vi "HardwareConfiguration.vi"() -> (3 "configured?":bool=TRUE)   [LabVIEW 2018]
uses:
  InstrControl/InstrumentSetup.vi
  globals/QC_RunInformation.vi
  InstrControl/InstrControl.lvclass
panel:
  in  "Matrix Configurations":bool
  in  "Defaults Multimeter":bool
  in  "Multimeter":enum32{"Keithley 2000"}(tab)
  in  "Range Value\n(0.1 - 100)":dbl=100.0 format="%#.2g"
  in  "Range":u16(ring) items=["Auto", "Manual"]
  in  "Function":u16(ring)=3 items=["AC Current", "DC Current", "AC Voltage", "DC Voltage", "2W-Resistance", "4W-Resistance", "Period", "Frequency", "Temperature", "Diode", "Continuity"]
  in  "Address KE2000":refnum<visa-resource-name>="GPIB0::19::INSTR"
  in  "Defaults LCR":bool
  in  "LCRs":T1(tab)=enum."HP4284A"
  in  "AC frequency [Hz]":i32=1000 format="%#.3p"
  in  "RC Configuration":u16(ring) items=["serial", "parallel"]
  in  "AC amplitude [V]":sgl=0.1
  in  "Address WK6440B":refnum<visa-resource-name>="GPIB0::6::INSTR"
  in  "Address WK6425":refnum<visa-resource-name>
  in  "AC amplitude [V] WK6425":sgl=0.1 caption="AC amplitude [V]"
  in  "RC Configuration WK6425":u16(ring) caption="RC Configuration" items=["serial", "parallel"]
  in  "AC frequency [Hz] WK6425":i32=1000 caption="AC frequency [Hz]" format="%#.3p"
  in  "Address HP4284A":refnum<visa-resource-name>="GPIB0::13::INSTR"
  in  "AC amplitude [V] HP4284A":sgl=0.1 caption="AC amplitude [V]"
  in  "AC frequency [Hz] HP4284A":i32=1000 caption="AC frequency [Hz]" format="%#.3p"
  in  "RC Configuration HP4284A":u16(ring)=6 caption="RC Configuration" items=["CPD", "CPQ", "CPG", "CPRP", "CSD", "CSQ", "CSRS", "LPQ", "LPD", "LPG", "LPRP", "LSD", "LSQ", "LSRS", "RX", "ZTD", "ZTR", "GB", "YTD", "YTR"]
  in  "Consider OC":bool
  in  "Consider SC":bool
  in  "VISA address":refnum<visa-resource-name>="COM24" caption="Arduino address"
  out "Programm uploaded?":string="Make sure programme is uploaded to Arduino Uno ->"
  in  "Blank Button":bool
  in  "Supplies":T2(tab)=enum."Keithley 237"
  in  "Current Limit [µA]":sgl=100.0
  in  "Address KE2410":refnum<visa-resource-name>="GPIB0::16::INSTR"
  in  "Address KE487":refnum<visa-resource-name>
  in  "Compliance":u16(ring) items=["20µA", "2mA"]
  in  "Range:":u16(ring) items=["Autorange", "2nA", "20nA", "200nA", "2 microAmp", "20 microAmp", "200 microAmp", "2 milliAmp"]
  in  "Current Limit":u16(ring)=1 items=["OFF", "ON"]
  in  "Address KE6517":refnum<visa-resource-name>
  in  "current compliance \nlevel [mA]":dbl=0.0001 format="%.4f"
  in  "compliance/measurement\nrange (auto:0)":u16(ring)=6 items=["auto / auto", "1 nA / 1.1 V", "10 nA / 11 V", "100 nA / 110 V", "0.001 mA / 110 V", "0.01 mA / 110 V", "0.1 mA / 110 V", "1 mA / 110 V", "10 mA / 110 V", "100 mA / 110 V"]
  in  "Address KE236":refnum<visa-resource-name>
  in  "Address KE237":refnum<visa-resource-name>="GPIB0::16::INSTR"
  in  "current compliance \nlevel [uA] K237":dbl=30.0 caption="current compliance\nlevel [uA]" format="%.4f"
  in  "compliance/measurement\nrange (auto:0) K237":u16(ring)=6 caption="compliance/measurement\nrange (auto:0)" items=["auto / auto", "1 nA / 1.1 V", "10 nA / 11 V", "100 nA / 110 V", "1 uA / 1100 V", "10 uA / *", "100 uA / *", "1 mA / *", "10 mA / *", "100 mA / *"]
  in  "Defaults Supply":bool
  in  "OK Button":bool
  # "Hardware Configuration"
  # "Multimeter Configuration"
  # "Supply Configuration"
  # "Arduino Configuration"
  # "LCR Configuration"
  # "(Only for initialisation)"
  # "(Only for initialisation)"
  # "(Only for initialisation)"
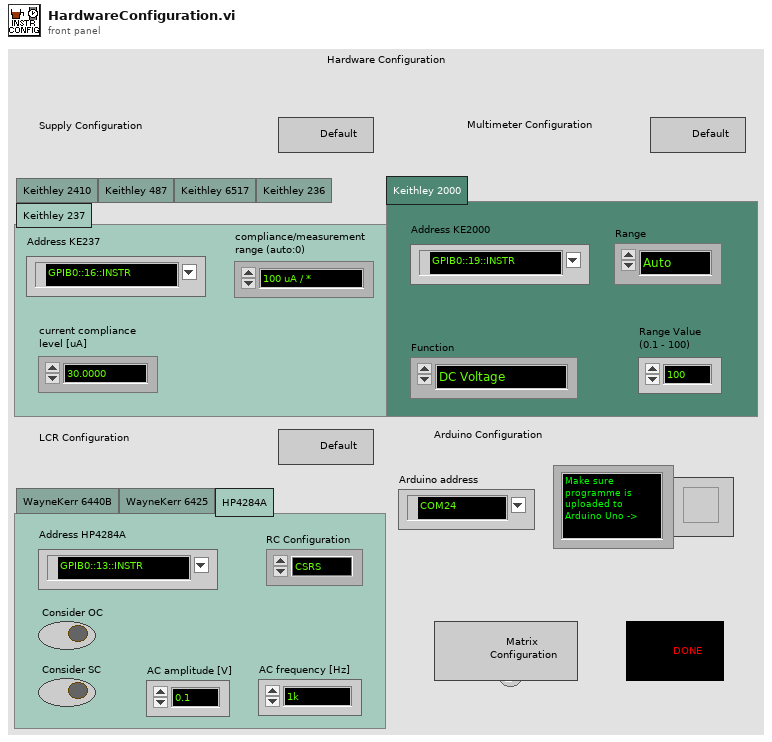
[diagram p1: front panel]
types:
  T1 = enum32{"WayneKerr 6440B", "WayneKerr 6425", "HP4284A"}
  T2 = enum32{"Keithley 2410", "Keithley 487", "Keithley 6517", "Keithley 236", "Keithley 237"}
  T3 = enum16{"CPD", "CPQ", "CPG", "CPRP", "CSD", "CSQ", "CSRS", "LPQ", "LPD", "LPG", "LPRP", "LSD", "LSQ", "LSRS", "RX", "ZTD", "ZTR", "GB", "YTD", "YTR"}
  T4 = cluster{"KE 2410":cluster{"Instrument name":string, "address":refnum<visa-resource-name>, "Instrument type":u16}, "KE 6517":cluster{"Instrument name":string, "address":refnum<visa-resource-name>, "Instrument type":u16}, "KE 487":cluster{"Instrument name":string, "address":refnum<visa-resource-name>, "Instrument type":u16}, "KE 236":cluster{"Instrument name":string, "address":refnum<visa-resource-name>, "Instrument type":u16}, "WK 6440B":cluster{"Instrument name":string, "address":refnum<visa-resource-name>, "Instrument type":u16}, "WK 6425":cluster{"Instrument name":string, "address":refnum<visa-resource-name>, "Instrument type":u16}, "Pickering Matrix":cluster{"Instrument name":string, "address":refnum<visa-resource-name>, "Instrument type":u16}, "KE 2000":cluster{"Instrument name":string, "address":refnum<visa-resource-name>, "Instrument type":u16}, "KE3706A Switching":cluster{"Instrument name":string, "address":refnum<visa-resource-name>, "Instrument type":u16}, "HP 4284A":cluster{"Instrument name":string, "address":refnum<visa-resource-name>, "Instrument type":u16}, "KE237":cluster{"Instrument name":string, "address":refnum<visa-resource-name>, "Instrument type":u16}}
  T5 = cluster{"VISA address":refnum<visa-resource-name>, "T sensor":enum16{"SHT", "DS"}, "Arduino":refnum<class "ArduinoControl.lvclass">}
  T6 = cluster{"Range":u16, "Range Value":dbl, "Function":u16, "KE2000":refnum<class "KE2000.lvclass">}
  T7 = cluster{"Current Limit":sgl, "KE2410":refnum<class "KE2410.lvclass">}
  T8 = cluster{"Compliance":u16, "Range:":u16, "KE487":refnum<class "KE487.lvclass">}
  T9 = cluster{"Current Limit":u16, "KE6517":refnum<class "KE6517.lvclass">}
  T10 = cluster{"current \ncompliance level":dbl, "compliance/\nmeasurement range (auto:0)":u16, "KE236":refnum<class "KE236.lvclass">}
  T11 = cluster{"current \ncompliance level":dbl, "compliance/\nmeasurement range (auto:0)":u16, "KE237":refnum<class "KE237.lvclass">}
  T12 = cluster{"Sensor Serial No.:":string, "Wafer Serial No.:":string, "Batch:":string, "Manufacturer:":string, "Device Category:":string, "Database Serial No.:":string, "Date Initiated:":string, "Time Initiated:":string, "Test":string, "Instruments used:":string, "Probeplan used:":string, "End of Run comment:":string, "User:":string}
  T13 = cluster{"RC Configuration":u16, "AC amplitude [V]":dbl, "AC frequency [Hz]":i32, "WK6440B":refnum<class "WK6440B.lvclass">}
  T14 = cluster{"RC Configuration":u16, "AC amplitude [V]":dbl, "AC frequency [Hz]":i32, "WK6425":refnum<class "WK6425.lvclass">}
  T15 = cluster{"RC Configuration":u16, "AC amplitude [V]":dbl, "Consider OC":bool, "Consider SC":bool, "AC frequency [Hz]":i32, "HP4284A":refnum<class "HP4284A.lvclass">}
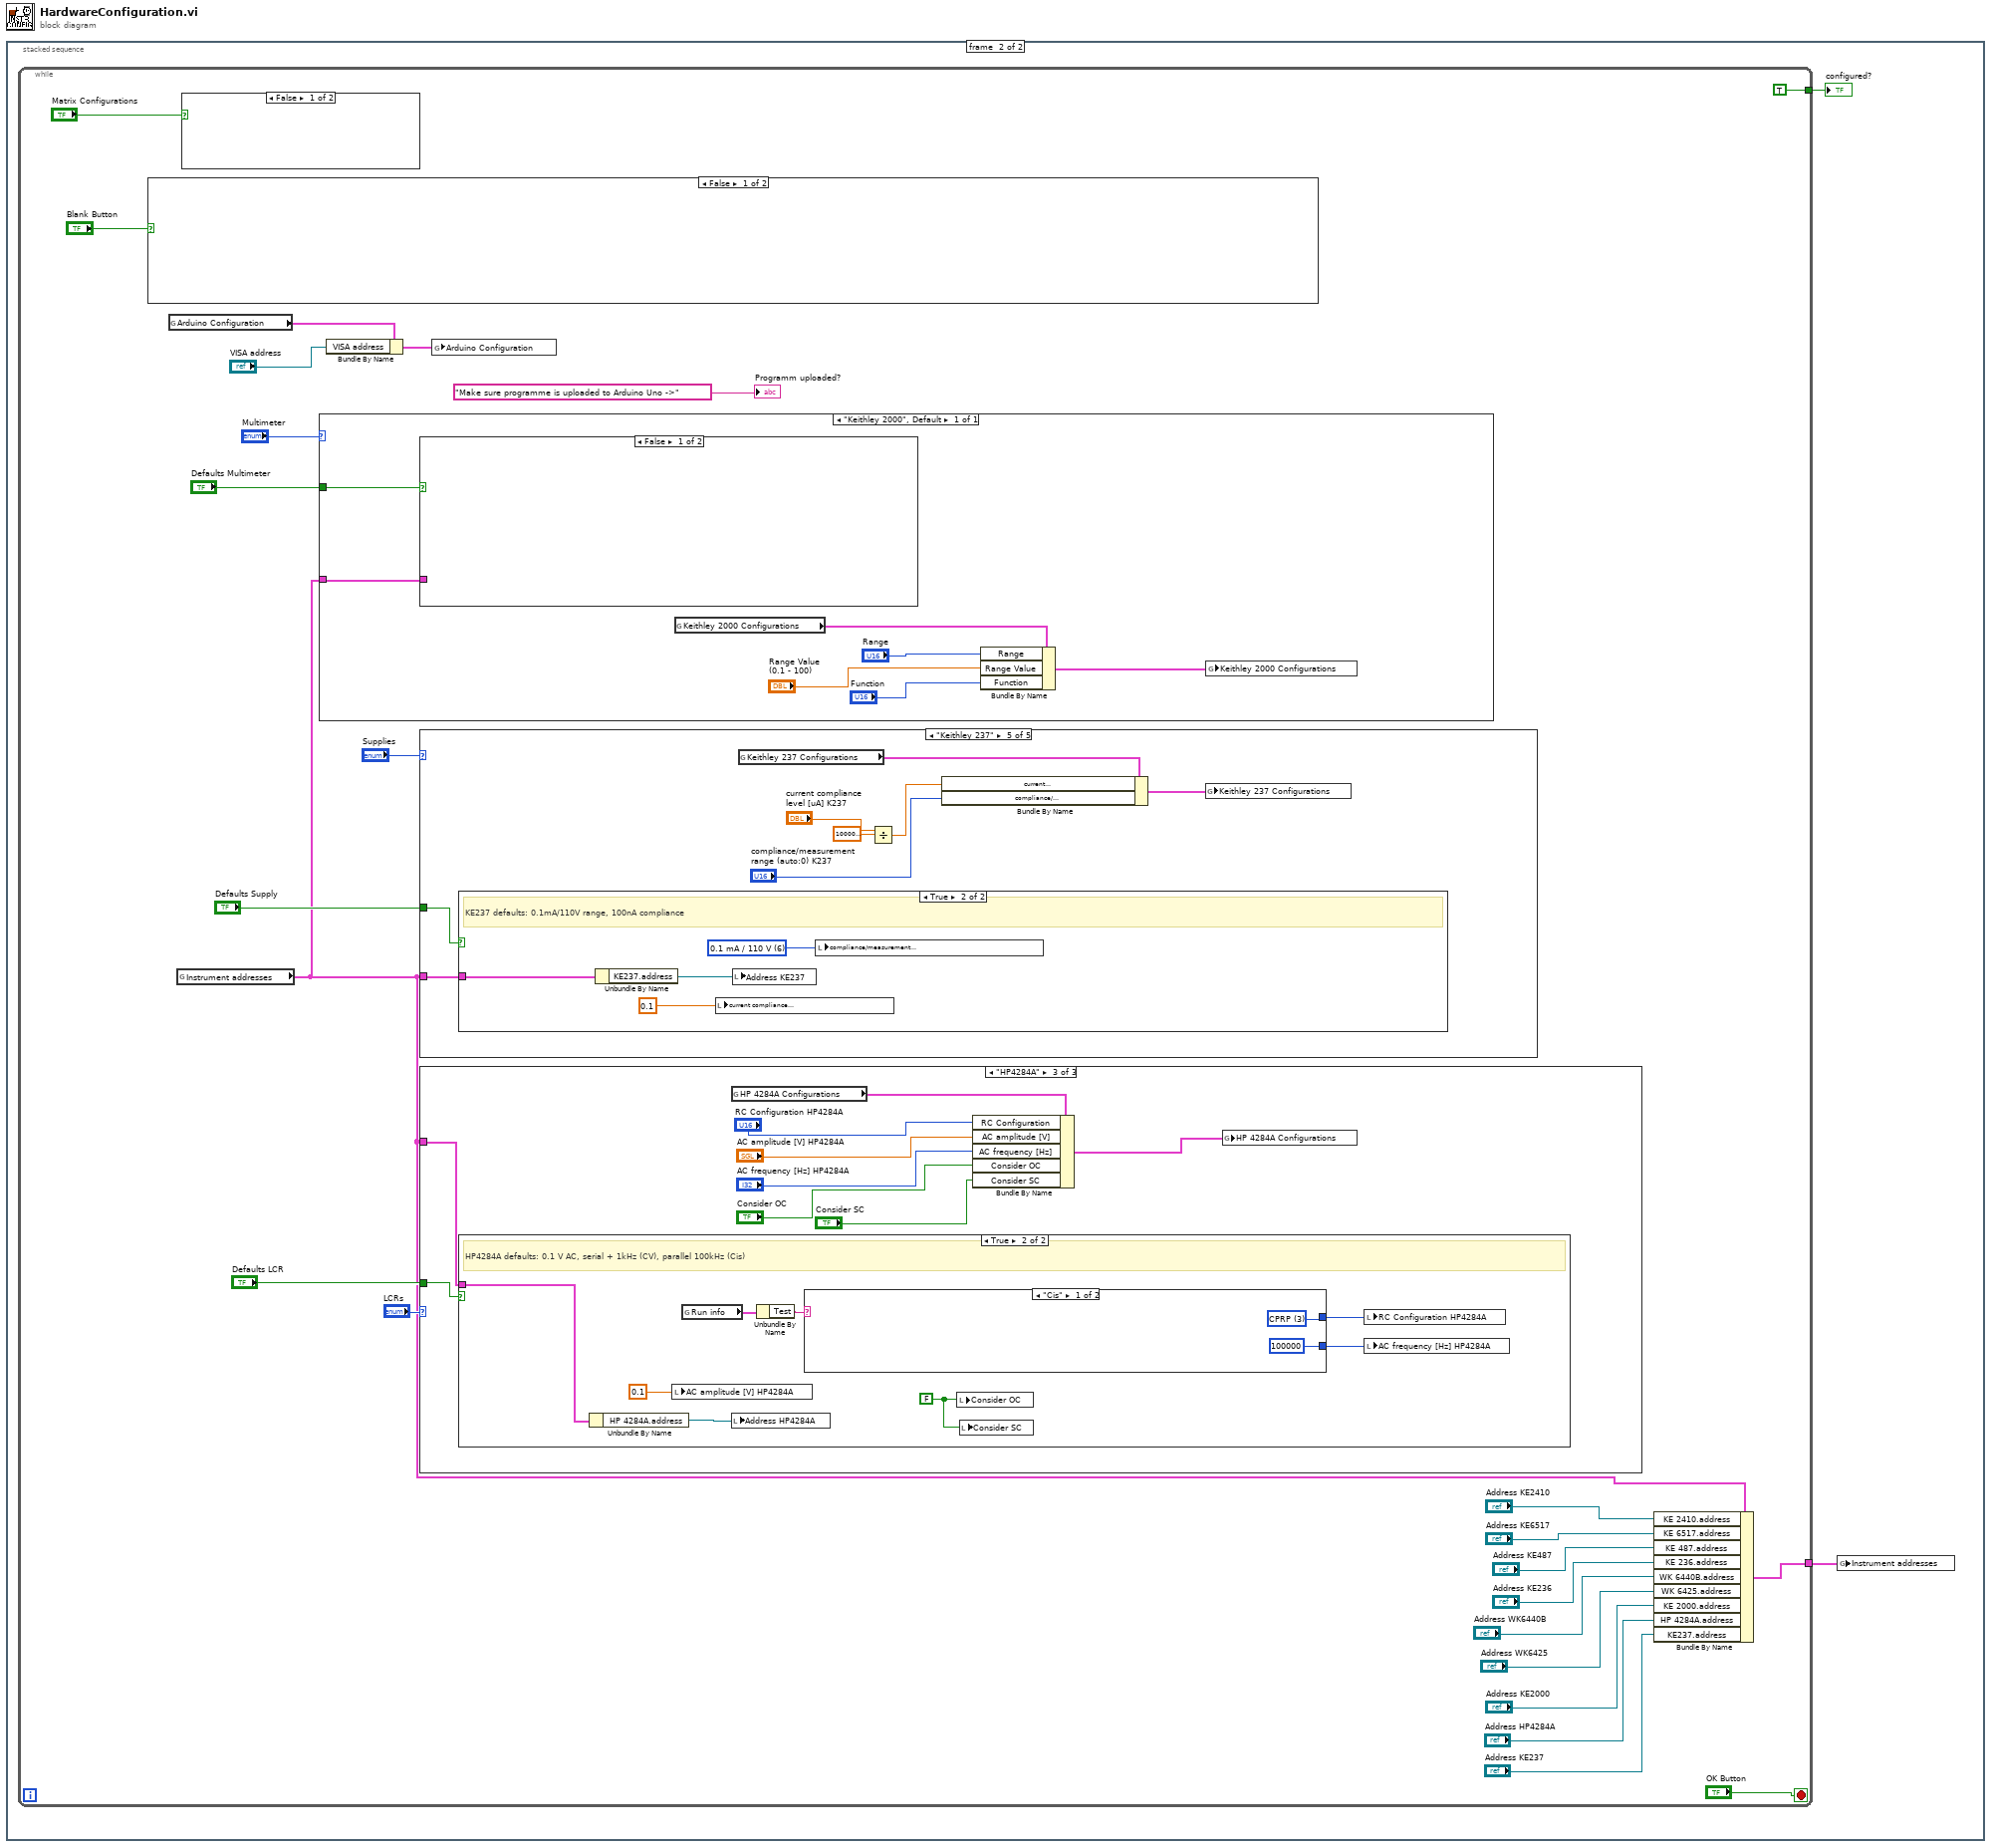
[diagram p0: block diagram]
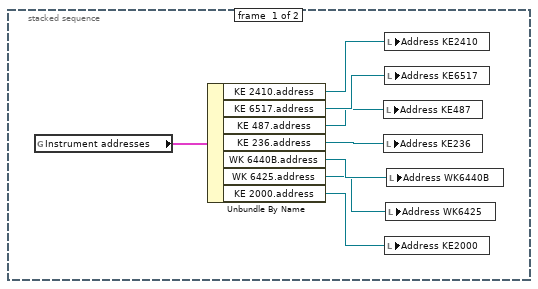
[diagram p2: hidden frame]
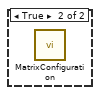
[diagram p3: hidden frame]
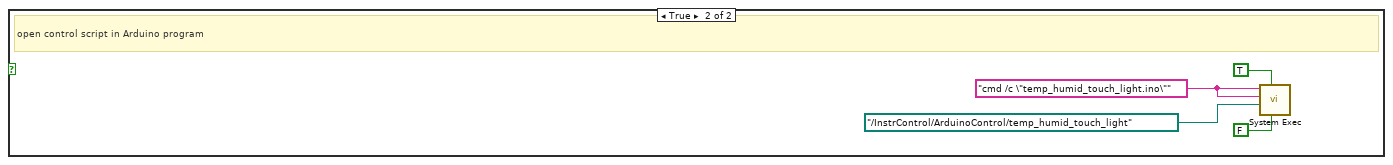
[diagram p4: hidden frame]
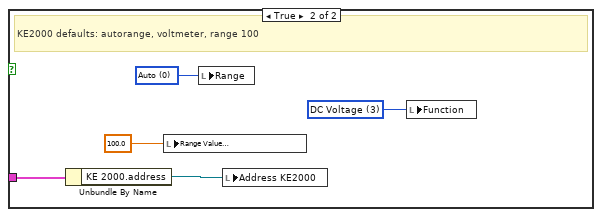
[diagram p5: hidden frame]
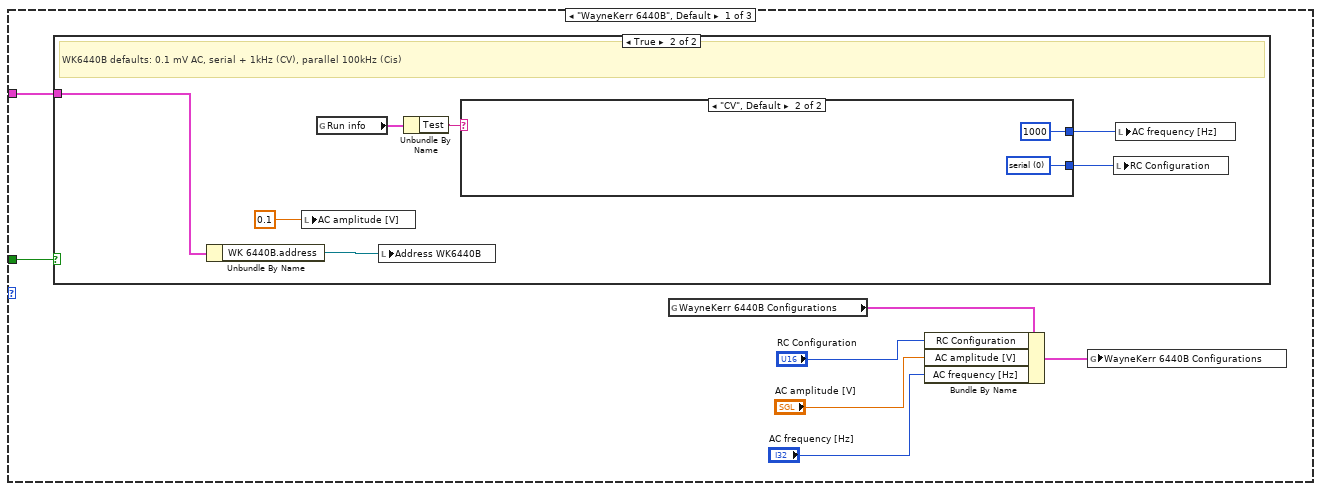
[diagram p6: hidden frame]
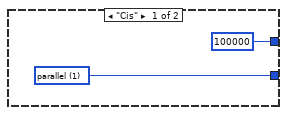
[diagram p8: hidden frame]
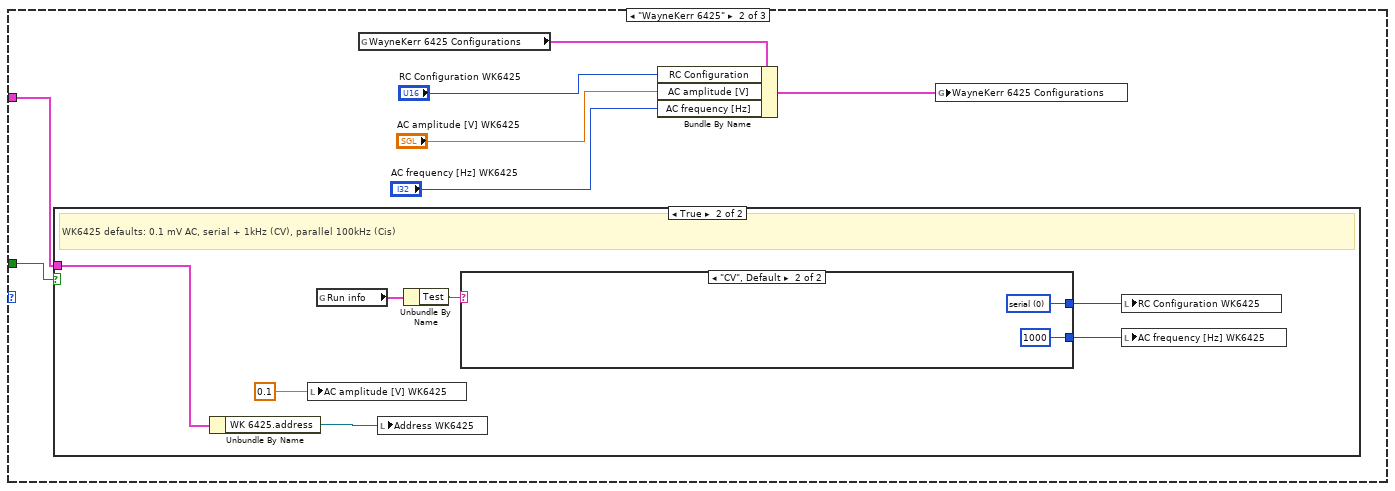
[diagram p9: hidden frame]
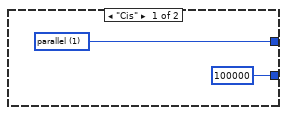
[diagram p11: hidden frame]
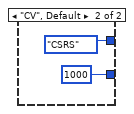
[diagram p13: hidden frame]
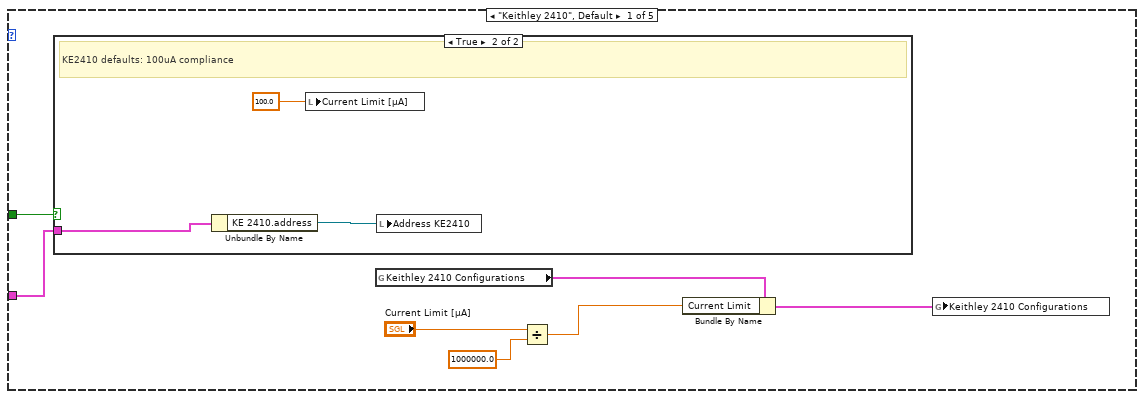
[diagram p14: hidden frame]
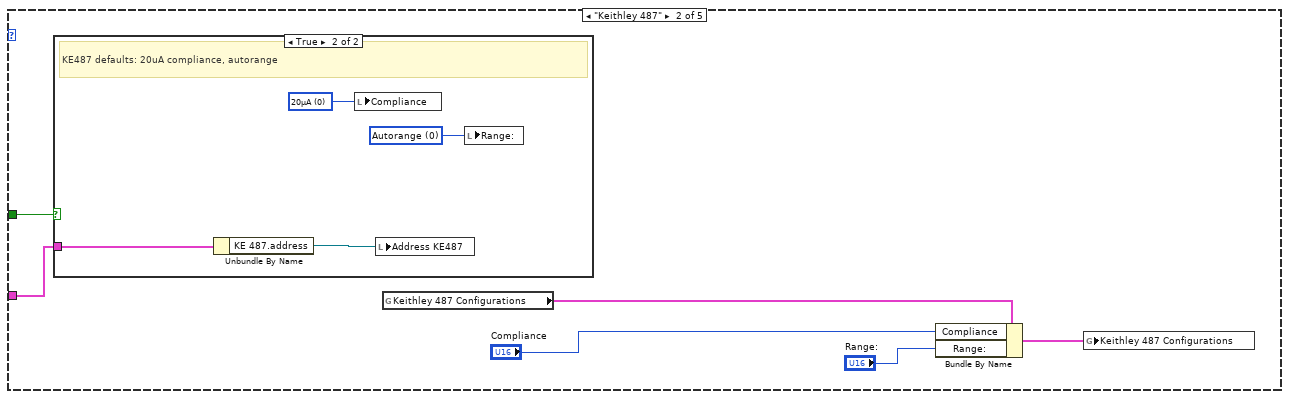
[diagram p16: hidden frame]
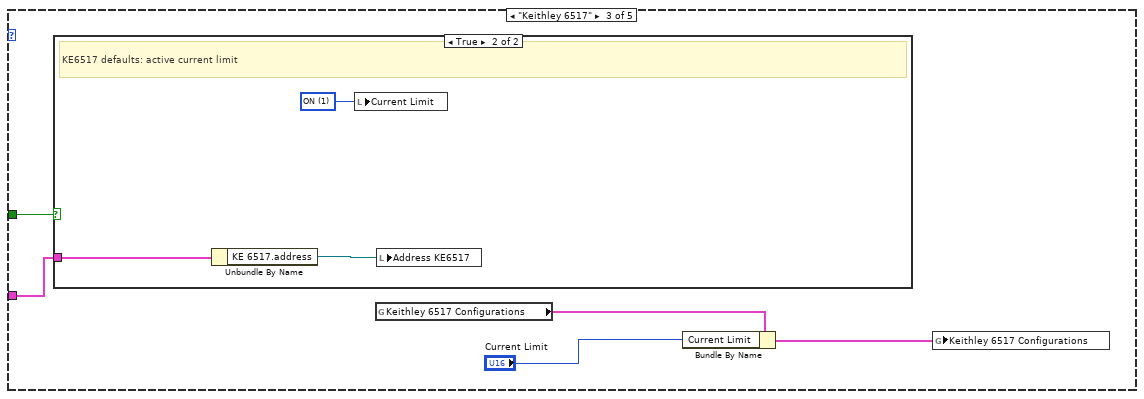
[diagram p18: hidden frame]
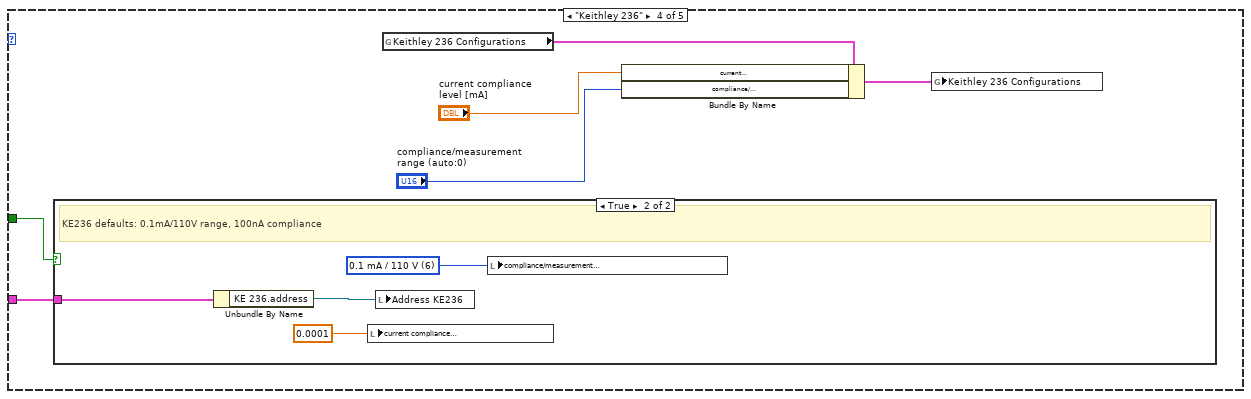
[diagram p20: hidden frame]
diagram:
  n1 = stacked-sequence {
    frame #0 {
      n2 = global read "InstrumentSetup.vi" "Instrument addresses"() -> (w8:T4)
      n3 = Unbundle By Name(w8) -> ("KE 2410.address"=w7:refnum<visa-resource-name>, "KE 6517.address"=w6:refnum<visa-resource-name>, "KE 487.address"=w5:refnum<visa-resource-name>, "KE 236.address"=w4:refnum<visa-resource-name>, "WK 6440B.address"=w3:refnum<visa-resource-name>, "WK 6425.address"=w2:refnum<visa-resource-name>, "KE 2000.address"=w1:refnum<visa-resource-name>)
      n4 = local write "Address KE487"(w5) -> ()
      n5 = local write "Address KE236"(w4) -> ()
      n6 = local write "Address KE2410"(w7) -> ()
      n7 = local write "Address KE6517"(w6) -> ()
      n8 = local write "Address KE2000"(w1) -> ()
      n9 = local write "Address WK6425"(w2) -> ()
      n10 = local write "Address WK6440B"(w3) -> ()
    }
    frame #1 {
      n11 = while {
        tunnel: [TRUE] -> w10
        tunnel: [w19] -> w9
        stop <- "OK Button" stop-if-true
        n12 = case shown="False" "Blank Button" {
          frame False {
          }
          frame True {
            w37 = "cmd /c \"temp_humid_touch_light.ino\""
            # "open control script in Arduino program"
            n13 = call <vilib>:"System Exec.vi"("run minimized? (F)"=FALSE, "wait until completion? (T)"=TRUE, "working directory"=path "../InstrControl/ArduinoControl/temp_humid_touch_light", "standard input"=w37, "command line"=w37) -> ()  [unwired: 3 in, 4 out]
          }
        }
        n14 = global read "InstrumentSetup.vi" "Arduino Configuration"() -> (w26:T5)
        n15 = global read "InstrumentSetup.vi" "Instrument addresses"() -> (w21:T4)
        n16 = case shown="False" "Matrix Configurations" {
          frame False {
          }
          frame True {
            n17 = call "MatrixConfiguration.vi"() -> ()  [unwired: 12 in]
          }
        }
        n18 = case shown="\"Keithley 2000\", Default" "Multimeter" {
          tunnel: "Defaults Multimeter" -> [w46]
          tunnel: w21 -> [w43]
          frame "Keithley 2000", Default {
            n19 = case shown="False" w46 {
              tunnel: w43 -> [_ w51]
              frame False {
              }
              frame True {
                w49 = u16 0 items=["Auto", "Manual"] ("Range")
                w50 = u16 3 items=["AC Current", "DC Current", "AC Voltage", "DC Voltage", "2W-Resistance", "4W-Resistance", "Period", "Frequency", "Temperature", "Diode", "Continuity"] ("Function")
                # "KE2000 defaults: autorange, voltmeter, range 100"
                n20 = Unbundle By Name(w51) -> ("KE 2000.address"=w47:refnum<visa-resource-name>)
                n21 = local write "Range Value\n(0.1 - 100)"(100.0 ("Range Value\n(0.1 - 100)")) -> ()
                n22 = local write "Range"(w49) -> ()
                n23 = local write "Address KE2000"(w47) -> ()
                n24 = local write "Function"(w50) -> ()
              }
            }
            n25 = global read "InstrumentSetup.vi" "Keithley 2000 Configurations"() -> (w45:T6)
            n26 = Bundle By Name(cluster=w45, "Range"="Range", "Range Value"="Range Value\n(0.1 - 100)", "Function"="Function") -> (w44:T6)
            n27 = global write "InstrumentSetup.vi" "Keithley 2000 Configurations"(w44) -> ()
          }
        }
        n28 = Bundle By Name(cluster=w26, "VISA address"="VISA address") -> (w25:T5)
        n29 = case shown="\"Keithley 237\"" "Supplies" {
          tunnel: "Defaults Supply" -> [w115 w124 w133 w142 w154]
          tunnel: w21 -> [w110 w121 w130 w139 w151]
          frame "Keithley 2410", Default {
            n30 = case shown="True" w115 {
              tunnel: w110 -> [_ w118]
              frame False {
              }
              frame True {
                # "KE2410 defaults: 100uA compliance"
                n31 = Unbundle By Name(w118) -> ("KE 2410.address"=w116:refnum<visa-resource-name>)
                n32 = local write "Current Limit [µA]"(100.0) -> ()
                n33 = local write "Address KE2410"(w116) -> ()
              }
            }
            n34 = global read "InstrumentSetup.vi" "Keithley 2410 Configurations"() -> (w114:T7)
            n35 = Divide(x="Current Limit [µA]", y=1000000.0) -> (x/y=w111:dbl)
            n36 = Bundle By Name(cluster=w114, "Current Limit"=w111) -> (w113:T7)
            n37 = global write "InstrumentSetup.vi" "Keithley 2410 Configurations"(w113) -> ()
          }
          frame "Keithley 487" {
            n38 = case shown="True" w124 {
              tunnel: w121 -> [_ w128]
              frame False {
              }
              frame True {
                w126 = u16 0 items=["Autorange", "2nA", "20nA", "200nA", "2 microAmp", "20 microAmp", "200 microAmp", "2 milliAmp"] ("Range:")
                w127 = u16 0 items=["20µA", "2mA"] ("Compliance")
                # "KE487 defaults: 20uA compliance, autorange"
                n39 = Unbundle By Name(w128) -> ("KE 487.address"=w125:refnum<visa-resource-name>)
                n40 = local write "Compliance"(w127) -> ()
                n41 = local write "Address KE487"(w125) -> ()
                n42 = local write "Range:"(w126) -> ()
              }
            }
            n43 = global read "InstrumentSetup.vi" "Keithley 487 Configurations"() -> (w123:T8)
            n44 = Bundle By Name(cluster=w123, "Compliance"="Compliance", "Range:"="Range:") -> (w122:T8)
            n45 = global write "InstrumentSetup.vi" "Keithley 487 Configurations"(w122) -> ()
          }
          frame "Keithley 6517" {
            n46 = case shown="True" w133 {
              tunnel: w130 -> [_ w136]
              frame False {
              }
              frame True {
                w135 = u16 1 items=["OFF", "ON"] ("Current Limit")
                # "KE6517 defaults: active current limit"
                n47 = Unbundle By Name(w136) -> ("KE 6517.address"=w134:refnum<visa-resource-name>)
                n48 = local write "Current Limit"(w135) -> ()
                n49 = local write "Address KE6517"(w134) -> ()
              }
            }
            n50 = global read "InstrumentSetup.vi" "Keithley 6517 Configurations"() -> (w132:T9)
            n51 = Bundle By Name(cluster=w132, "Current Limit"="Current Limit") -> (w131:T9)
            n52 = global write "InstrumentSetup.vi" "Keithley 6517 Configurations"(w131) -> ()
          }
          frame "Keithley 236" {
            n53 = case shown="True" w142 {
              tunnel: w139 -> [_ w146]
              frame False {
              }
              frame True {
                w144 = u16 6 items=["auto / auto", "1 nA / 1.1 V", "10 nA / 11 V", "100 nA / 110 V", "0.001 mA / 110 V", "0.01 mA / 110 V", "0.1 mA / 110 V", "1 mA / 110 V", "10 mA / 110 V", "100 mA / 110 V"] ("compliance/\nmeasurement range (auto:0)")
                # "KE236 defaults: 0.1mA/110V range, 100nA compliance"
                n54 = Unbundle By Name(w146) -> ("KE 236.address"=w143:refnum<visa-resource-name>)
                n55 = local write "current compliance \nlevel [mA]"(0.0001 ("current \ncompliance level")) -> ()
                n56 = local write "Address KE236"(w143) -> ()
                n57 = local write "compliance/measurement\nrange (auto:0)"(w144) -> ()
              }
            }
            n58 = global read "InstrumentSetup.vi" "Keithley 236 Configurations"() -> (w140:T10)
            n59 = Bundle By Name(cluster=w140, "current \ncompliance level"="current compliance \nlevel [mA]", "compliance/\nmeasurement range (auto:0)"="compliance/measurement\nrange (auto:0)") -> (w141:T10)
            n60 = global write "InstrumentSetup.vi" "Keithley 236 Configurations"(w141) -> ()
          }
          frame "Keithley 237" {
            n61 = case shown="True" w154 {
              tunnel: w151 -> [_ w158]
              frame False {
              }
              frame True {
                w157 = u16 6 items=["auto / auto", "1 nA / 1.1 V", "10 nA / 11 V", "100 nA / 110 V", "0.001 mA / 110 V", "0.01 mA / 110 V", "0.1 mA / 110 V", "1 mA / 110 V", "10 mA / 110 V", "100 mA / 110 V"] ("compliance/\nmeasurement range (auto:0)")
                # "KE237 defaults: 0.1mA/110V range, 100nA compliance"
                n62 = Unbundle By Name(w158) -> ("KE237.address"=w156:refnum<visa-resource-name>)
                n63 = local write "current compliance \nlevel [uA] K237"(0.1 ("current \ncompliance level")) -> ()
                n64 = local write "Address KE237"(w156) -> ()
                n65 = local write "compliance/measurement\nrange (auto:0) K237"(w157) -> ()
              }
            }
            n66 = global read "InstrumentSetup.vi" "Keithley 237 Configurations"() -> (w152:T11)
            n67 = Divide(x="current compliance \nlevel [uA] K237", y=1000000.0) -> (x/y=w148:dbl)
            n68 = Bundle By Name(cluster=w152, "current \ncompliance level"=w148, "compliance/\nmeasurement range (auto:0)"="compliance/measurement\nrange (auto:0) K237") -> (w153:T11)
            n69 = global write "InstrumentSetup.vi" "Keithley 237 Configurations"(w153) -> ()
          }
        }
        n70 = case shown="\"HP4284A\"" "LCRs" {
          tunnel: "Defaults LCR" -> [w56 w74 w94]
          tunnel: w21 -> [w55 w73 w93]
          frame "WayneKerr 6440B", Default {
            n71 = case shown="True" w56 {
              tunnel: w55 -> [_ w65]
              frame False {
              }
              frame True {
                # "WK6440B defaults: 0.1 mV AC, serial + 1kHz (CV), parallel 100kHz (Cis)"
                n72 = Unbundle By Name(w65) -> ("WK 6440B.address"=w59:refnum<visa-resource-name>)
                n73 = local write "AC amplitude [V]"(0.1) -> ()
                n74 = global read "QC_RunInformation.vi" "Run info"() -> (w61:T12)
                n75 = local write "Address WK6440B"(w59) -> ()
                n76 = Unbundle By Name(w61) -> ("Test"=w60:string)
                n77 = case shown="\"CV\", Default" w60 {
                  tunnel: [w67 w69] -> w63
                  tunnel: [100000 1000] -> w62
                  frame "Cis" {
                    w67 = u16 1 items=["serial", "parallel"] ("RC Configuration")
                  }
                  frame "CV", Default {
                    w69 = u16 0 items=["serial", "parallel"] ("RC Configuration")
                  }
                }
                n78 = local write "RC Configuration"(w63) -> ()
                n79 = local write "AC frequency [Hz]"(w62) -> ()
              }
            }
            n80 = global read "InstrumentSetup.vi" "WayneKerr 6440B Configurations"() -> (w58:T13)
            n81 = Bundle By Name(cluster=w58, "RC Configuration"="RC Configuration", "AC amplitude [V]"="AC amplitude [V]", "AC frequency [Hz]"="AC frequency [Hz]") -> (w57:T13)
            n82 = global write "InstrumentSetup.vi" "WayneKerr 6440B Configurations"(w57) -> ()
          }
          frame "WayneKerr 6425" {
            n83 = case shown="True" w74 {
              tunnel: w73 -> [_ w83]
              frame False {
              }
              frame True {
                # "WK6425 defaults: 0.1 mV AC, serial + 1kHz (CV), parallel 100kHz (Cis)"
                n84 = Unbundle By Name(w83) -> ("WK 6425.address"=w77:refnum<visa-resource-name>)
                n85 = local write "AC amplitude [V] WK6425"(0.1) -> ()
                n86 = global read "QC_RunInformation.vi" "Run info"() -> (w79:T12)
                n87 = local write "Address WK6425"(w77) -> ()
                n88 = Unbundle By Name(w79) -> ("Test"=w78:string)
                n89 = case shown="\"CV\", Default" w78 {
                  tunnel: [w85 w87] -> w81
                  tunnel: [100000 1000] -> w80
                  frame "Cis" {
                    w85 = u16 1 items=["serial", "parallel"] ("RC Configuration")
                  }
                  frame "CV", Default {
                    w87 = u16 0 items=["serial", "parallel"] ("RC Configuration")
                  }
                }
                n90 = local write "RC Configuration WK6425"(w81) -> ()
                n91 = local write "AC frequency [Hz] WK6425"(w80) -> ()
              }
            }
            n92 = global read "InstrumentSetup.vi" "WayneKerr 6425 Configurations"() -> (w76:T14)
            n93 = Bundle By Name(cluster=w76, "RC Configuration"="RC Configuration WK6425", "AC amplitude [V]"="AC amplitude [V] WK6425", "AC frequency [Hz]"="AC frequency [Hz] WK6425") -> (w75:T14)
            n94 = global write "InstrumentSetup.vi" "WayneKerr 6425 Configurations"(w75) -> ()
          }
          frame "HP4284A" {
            n95 = case shown="True" w94 {
              tunnel: w93 -> [_ w104]
              frame False {
              }
              frame True {
                w97 = FALSE
                # "HP4284A defaults: 0.1 V AC, serial + 1kHz (CV), parallel 100kHz (Cis)"
                n96 = Unbundle By Name(w104) -> ("HP 4284A.address"=w98:refnum<visa-resource-name>)
                n97 = local write "AC amplitude [V] HP4284A"(0.1) -> ()
                n98 = global read "QC_RunInformation.vi" "Run info"() -> (w100:T12)
                n99 = local write "Address HP4284A"(w98) -> ()
                n100 = Unbundle By Name(w100) -> ("Test"=w99:string)
                n101 = case shown="\"Cis\"" w99 {
                  tunnel: [w105 T3."CSRS" ("RC Configuration HP4284A")] -> w102
                  tunnel: [100000 1000] -> w101
                  frame "Cis" {
                    w105 = u16 3 items=["CPD", "CPQ", "CPG", "CPRP", "CSD", "CSQ", "CSRS", "LPQ", "LPD", "LPG", "LPRP", "LSD", "LSQ", "LSRS", "RX", "ZTD", "ZTR", "GB", "YTD", "YTR"] ("RC Configuration HP4284A")
                  }
                  frame "CV", Default {
                  }
                }
                n102 = local write "Consider OC"(w97) -> ()
                n103 = local write "Consider SC"(w97) -> ()
                n104 = local write "RC Configuration HP4284A"(w102) -> ()
                n105 = local write "AC frequency [Hz] HP4284A"(w101) -> ()
              }
            }
            n106 = global read "InstrumentSetup.vi" "HP 4284A Configurations"() -> (w96:T15)
            n107 = Bundle By Name(cluster=w96, "RC Configuration"="RC Configuration HP4284A", "AC amplitude [V]"="AC amplitude [V] HP4284A", "AC frequency [Hz]"="AC frequency [Hz] HP4284A", "Consider OC"="Consider OC", "Consider SC"="Consider SC") -> (w95:T15)
            n108 = global write "InstrumentSetup.vi" "HP 4284A Configurations"(w95) -> ()
          }
        }
        n109 = global write "InstrumentSetup.vi" "Arduino Configuration"(w25) -> ()
        n110 = Bundle By Name(cluster=w21, "KE 2410.address"="Address KE2410", "KE 6517.address"="Address KE6517", "KE 487.address"="Address KE487", "KE 236.address"="Address KE236", "WK 6440B.address"="Address WK6440B", "WK 6425.address"="Address WK6425", "KE 2000.address"="Address KE2000", "HP 4284A.address"="Address HP4284A", "KE237.address"="Address KE237") -> (w19:T4)
        "Programm uploaded?" <- "Make sure programme is uploaded to Arduino Uno ->"
      }
      "configured?" <- w10
      n111 = global write "InstrumentSetup.vi" "Instrument addresses"(w9) -> ()
    }
  }
